vi "Video read with led for drums.vi"() -> ()   [LabVIEW 2009]
uses:
  <vilib>/vision/Image Controls.llb/IMAQ Image.ctl
  <vilib>/Instr/_visa.llb/VISA Configure Serial Port (Instr).vi
  <vilib>/Analysis/3filter.llb/Filter Passband Type.ctl
  <vilib>/Analysis/3filter.llb/Butterworth Filter (DBL).vi
  <vilib>/vision/NI_Vision_Development_Module.lvlib
  <vilib>/Analysis/NI_AALBase.lvlib
panel:
  in  "Mask":T1 {"Contours"."Type" items=["No Selection", "Point", "Line", "Rectangle", "Oval", "Polygon", "Freehand Region", "Annulus", "Unused2", "Unused3", "Broken Line", "Freehand Line", "Rotated Rectangle"]}
  out "Image 2":T2(plugin-control)
  out "Red Line":T1={"Global Rectangle"=[300, 297, 320, 380], "Contours"=[{"ID"=enum."External", "Type"=2, "Coordinates"=[300, 379, 319, 297]}]} {"Contours"."Type" items=["No Selection", "Point", "Line", "Rectangle", "Oval", "Polygon", "Freehand Region", "Annulus", "Unused2", "Unused3", "Broken Line", "Freehand Line", "Rotated Rectangle"]}
  in  "Red Line":T1={"Global Rectangle"=[300, 297, 320, 380], "Contours"=[{"ID"=enum."External", "Type"=2, "Coordinates"=[300, 379, 319, 297]}]} {"Contours"."Type" items=["No Selection", "Point", "Line", "Rectangle", "Oval", "Polygon", "Freehand Region", "Annulus", "Unused2", "Unused3", "Broken Line", "Freehand Line", "Rotated Rectangle"]}
  out "Waveform Red":dbl[](graph)
  out "LED Red":bool
  in  "sampling 4":dbl=1.0 format="%0.2f"
  in  "high 4":dbl=60.0 format="%0.2f"
  in  "low  4":dbl=0.12500000000000006 format="%0.4f"
  out "Green Line":T1={"Global Rectangle"=[406, 309, 423, 383], "Contours"=[{"ID"=enum."External", "Type"=2, "Coordinates"=[422, 382, 406, 309]}]} {"Contours"."Type" items=["No Selection", "Point", "Line", "Rectangle", "Oval", "Polygon", "Freehand Region", "Annulus", "Unused2", "Unused3", "Broken Line", "Freehand Line", "Rotated Rectangle"]}
  in  "Blue Line":T1={"Global Rectangle"=[374, 278, 383, 377], "Contours"=[{"ID"=enum."External", "Type"=2, "Coordinates"=[382, 376, 374, 278]}]} {"Contours"."Type" items=["No Selection", "Point", "Line", "Rectangle", "Oval", "Polygon", "Freehand Region", "Annulus", "Unused2", "Unused3", "Broken Line", "Freehand Line", "Rotated Rectangle"]}
  in  "Green Line":T1={"Global Rectangle"=[406, 309, 423, 383], "Contours"=[{"ID"=enum."External", "Type"=2, "Coordinates"=[422, 382, 406, 309]}]} {"Contours"."Type" items=["No Selection", "Point", "Line", "Rectangle", "Oval", "Polygon", "Freehand Region", "Annulus", "Unused2", "Unused3", "Broken Line", "Freehand Line", "Rotated Rectangle"]}
  in  "low  3":dbl=0.12500000000000006 format="%0.4f"
  out "Waveform Green":dbl[](graph)
  out "LED Green":bool
  in  "sampling 3":dbl=1.0 format="%0.2f"
  in  "high 3":dbl=60.0 format="%0.2f"
  in  "Yellow Line":T1={"Global Rectangle"=[342, 292, 349, 377], "Contours"=[{"ID"=enum."External", "Type"=2, "Coordinates"=[342, 376, 348, 292]}]} {"Contours"."Type" items=["No Selection", "Point", "Line", "Rectangle", "Oval", "Polygon", "Freehand Region", "Annulus", "Unused2", "Unused3", "Broken Line", "Freehand Line", "Rotated Rectangle"]}
  out "Blue Line":T1={"Global Rectangle"=[168, 264, 180, 378], "Contours"=[{"ID"=enum."External", "Type"=2, "Coordinates"=[168, 377, 179, 264]}]} {"Contours"."Type" items=["No Selection", "Point", "Line", "Rectangle", "Oval", "Polygon", "Freehand Region", "Annulus", "Unused2", "Unused3", "Broken Line", "Freehand Line", "Rotated Rectangle"]}
  out "cluster":T3
  in  "baud rate (9600)":u32=9600
  in  "VISA resource name":refnum<visa-resource-name>
  out "number":u32
  out "decimal integer string":string
  out "Image Dst Out":T2
  out "Yellow Line":T1={"Global Rectangle"=[243, 262, 261, 384], "Contours"=[{"ID"=enum."External", "Type"=2, "Coordinates"=[260, 383, 243, 262]}]} {"Contours"."Type" items=["No Selection", "Point", "Line", "Rectangle", "Oval", "Polygon", "Freehand Region", "Annulus", "Unused2", "Unused3", "Broken Line", "Freehand Line", "Rotated Rectangle"]}
  in  "low  2":dbl=0.12500000000000006 format="%0.4f"
  in  "high 2":dbl=60.0 format="%0.2f"
  in  "sampling 2":dbl=1.0 format="%0.2f"
  out "LED Yellow":bool
  out "Waveform Yellow":dbl[](graph)
  in  "playtime":dbl=30.0
  out "Frame Number":i32
  in  "Frame Start":i32=2400
  out "LED BLUE":bool
  in  "low":dbl=0.12500000000000006 format="%0.4f"
  out "Waveform Blue":dbl[](graph)
  in  "high":dbl=60.0 format="%0.2f"
  in  "sampling":dbl=1.0 format="%0.2f"
  in  "stop":bool
  in  "AVI Path":path
  # "BLUE"
  # "YELLOW"
  # "GREEN"
  # "RED"
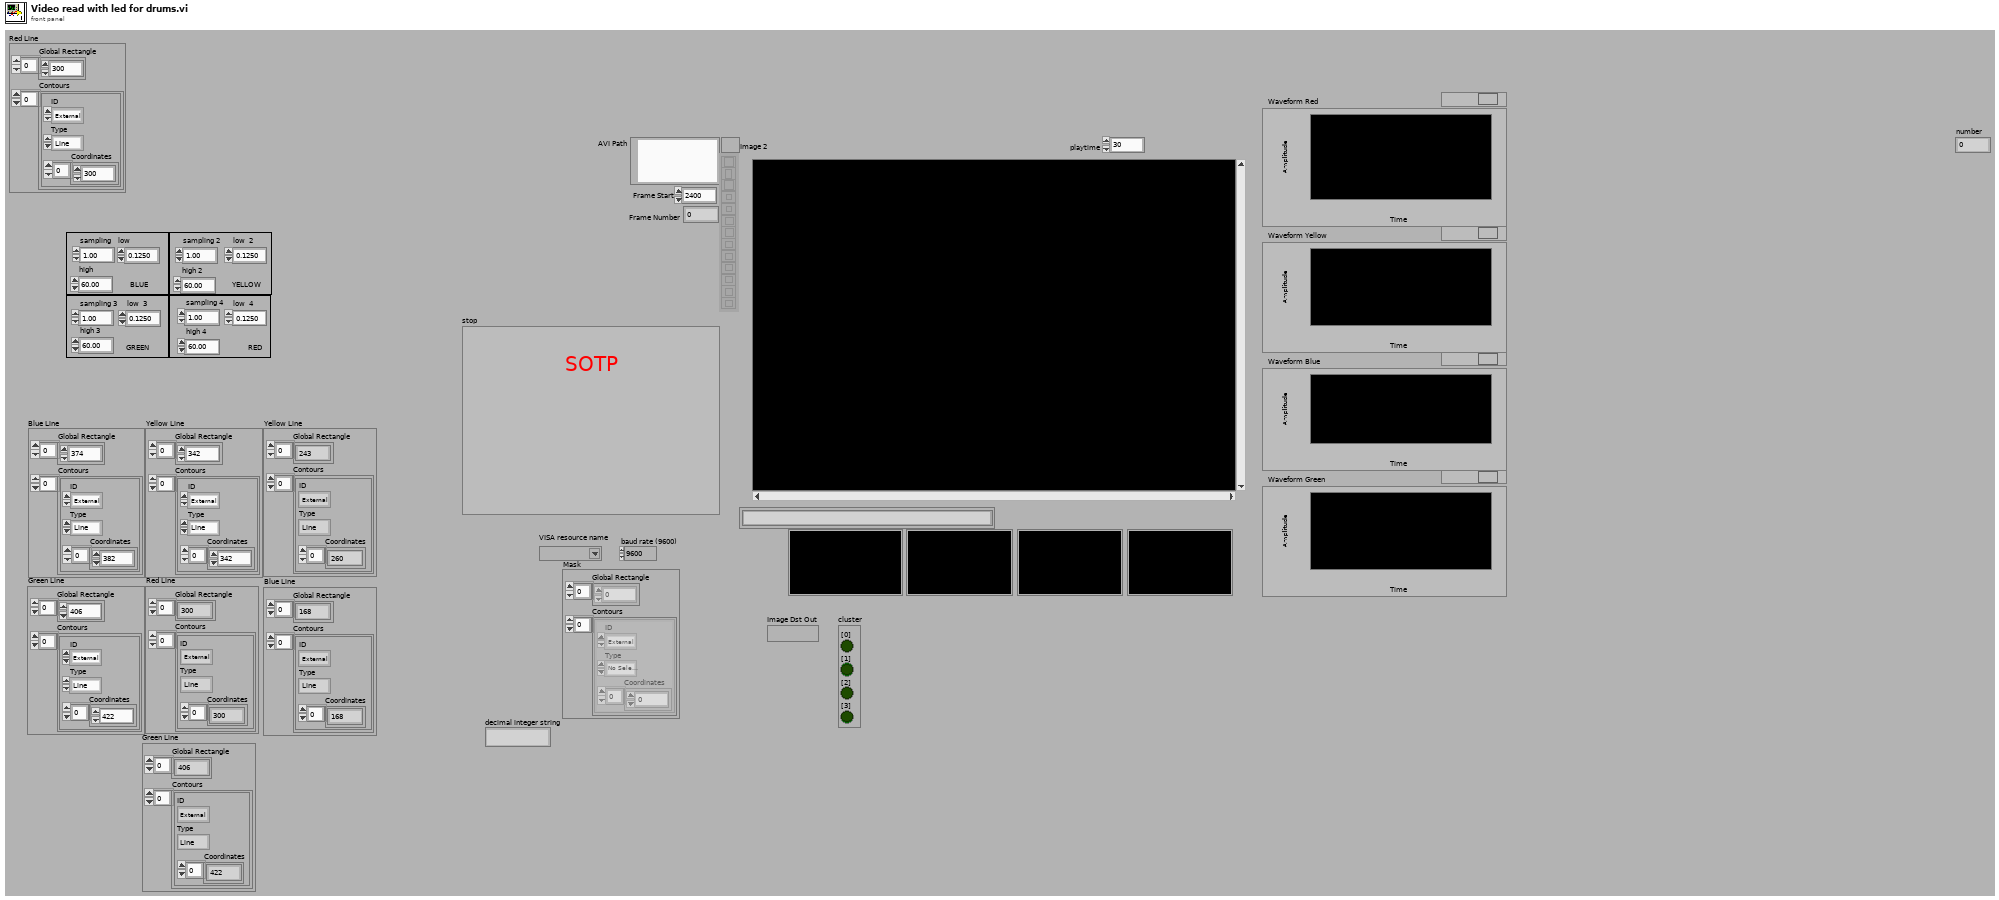
[diagram p1: front panel]
types:
  T1 = cluster{"Global Rectangle":i32[], "Contours":cluster{"ID":enum32{"External", "Internal"}, "Type":u32, "Coordinates":i32[]}[]}
  T2 = typedef "IMAQ Image.ctl" = refnum<image>
  T3 = cluster{"[0]":bool, "[1]":bool, "[2]":bool, "[3]":bool, "[4]":bool, "[5]":bool, "[6]":bool, "[7]":bool, "[8]":bool}
  T4 = typedef "NI_AALBase.lvlib/Filter Passband Type.ctl" = enum32{"Lowpass", "Highpass", "Bandpass", "Bandstop"}
  T5 = cluster{"Left":i32, "Top":i32, "Right":i32, "Bottom":i32}
  T6 = typedef "Image Type" = u32
  T7 = typedef "AviRefnum.ctl" = refnum<k1>
  T8 = cluster{"ID":enum32{"External", "Internal"}, "Type":u32, "Coordinates":i32[]}[]
  T9 = cluster{"ID":enum32{"External", "Internal"}, "Type":u32, "Coordinates":i32[]}
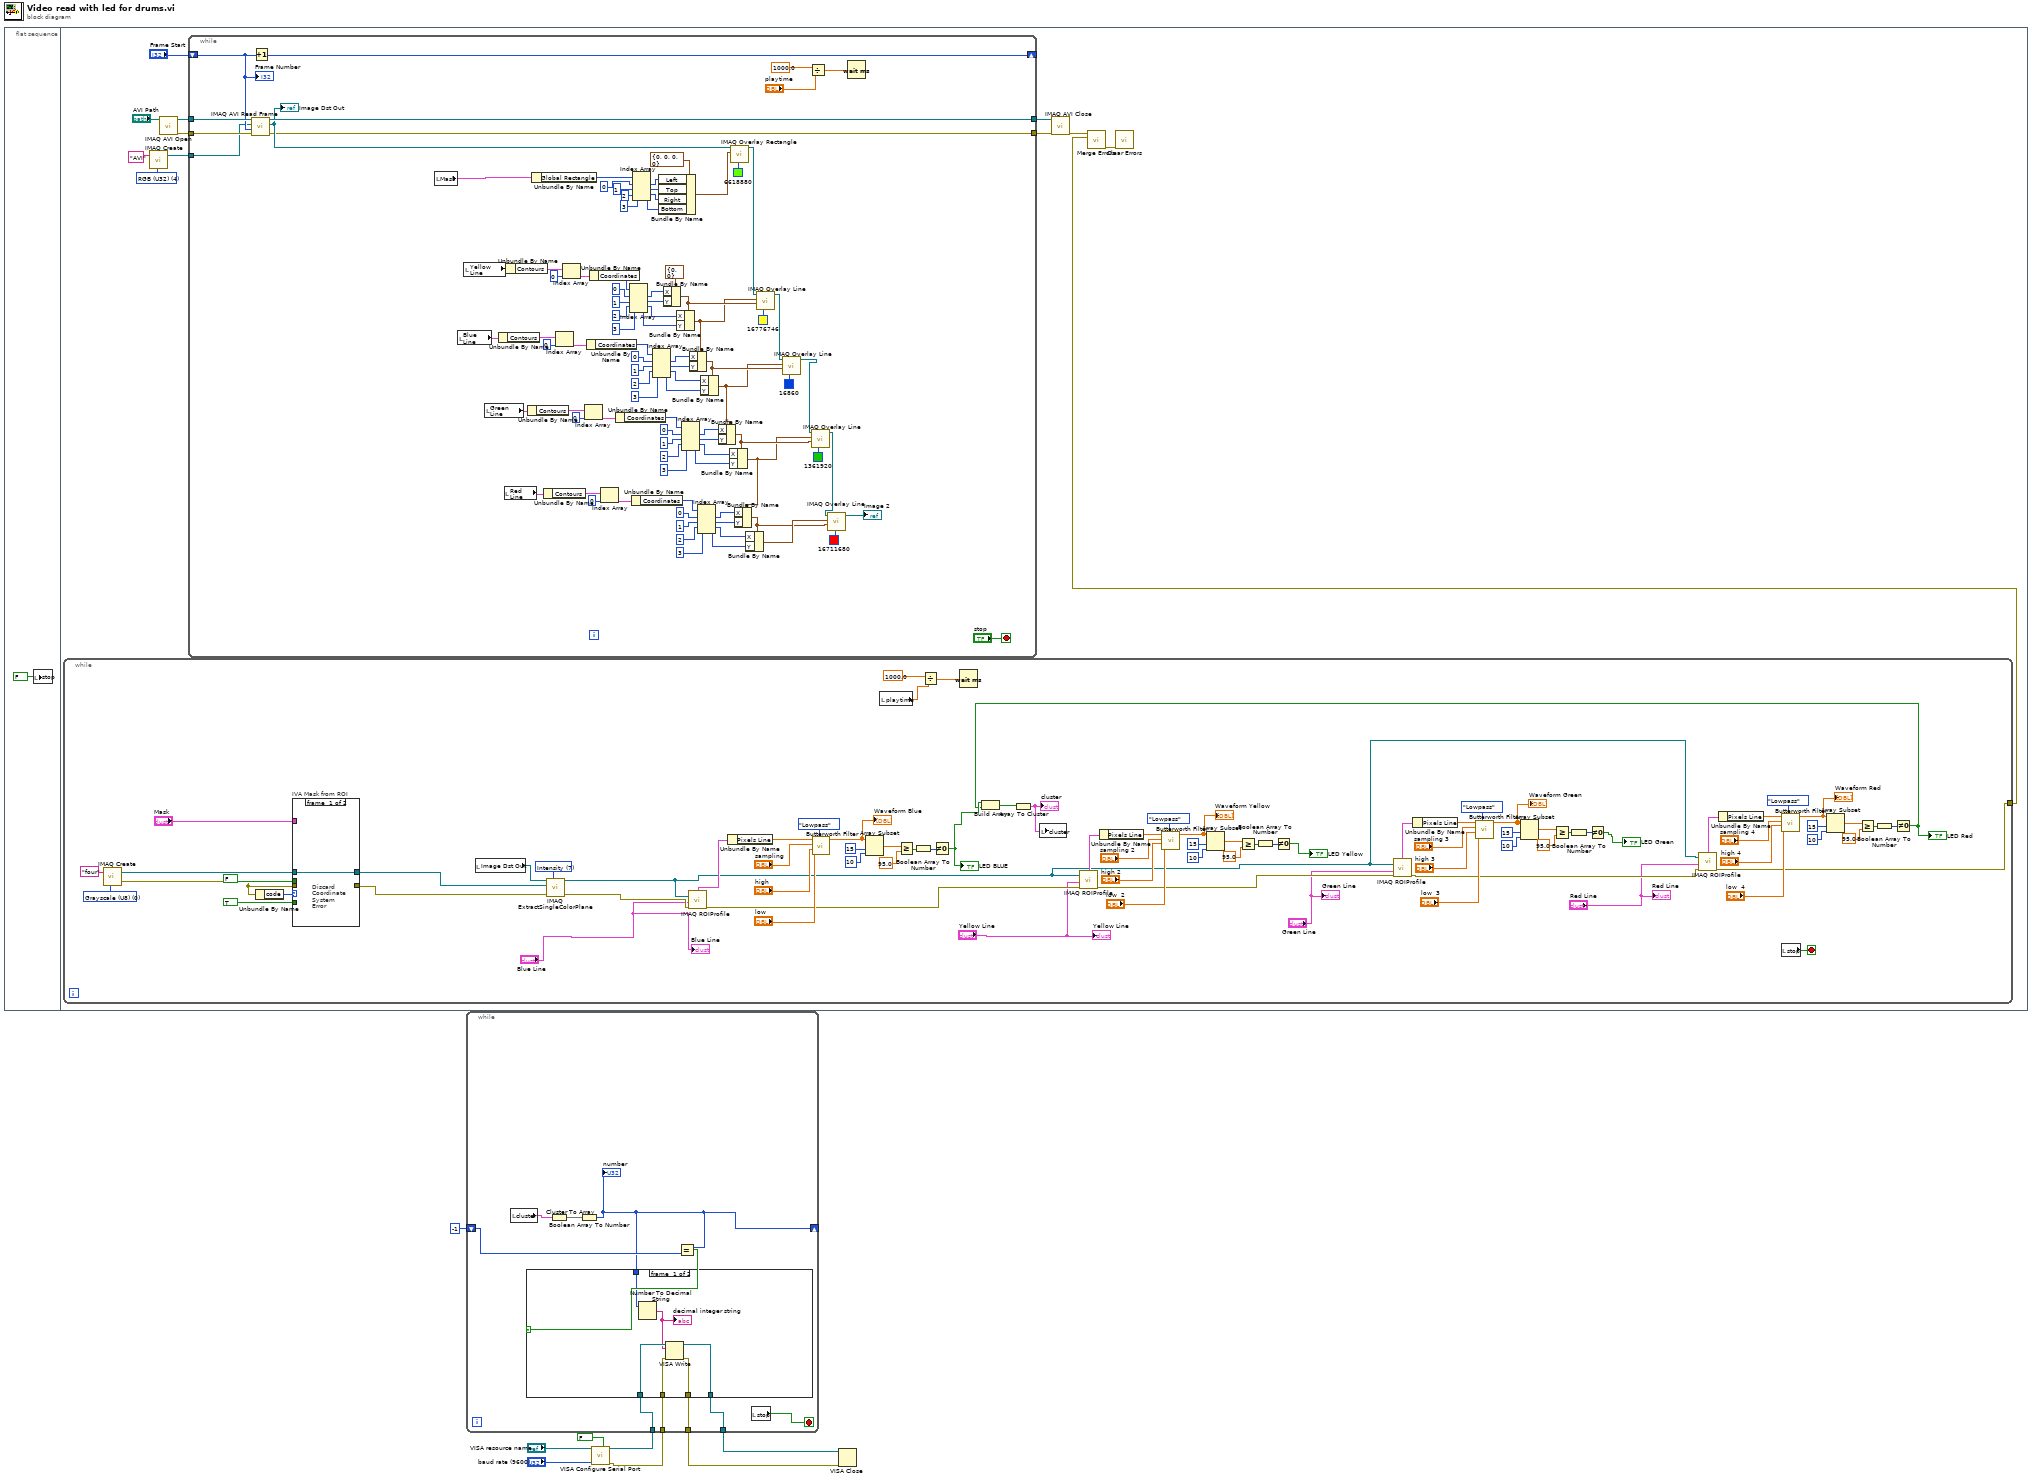
[diagram p0: block diagram]
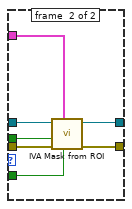
[diagram p3: hidden frame]
diagram:
  n1 = flat-sequence {
    frame #0 {
      n2 = local write "stop"(FALSE ("stop")) -> ()
    }
    frame #1 {
      w13 = T6 4 items=["Grayscale (U8)", "Grayscale (I16)", "Grayscale (SGL)", "Complex (CSG)", "RGB (U32)", "HSL (U32)", "RGB (U64)", "Grayscale (U16)"] ("Image Type")
      n3 = while {
        tunnel: [w34] -> w10
        stop <- w104 stop-if-true
        w75 = T6 0 items=["Grayscale (U8)", "Grayscale (I16)", "Grayscale (SGL)", "Complex (CSG)", "RGB (U32)", "HSL (U32)", "RGB (U64)", "Grayscale (U16)"] ("Image Type")
        w105 = 7 items=["Red", "Green", "Blue", "Hue", "Saturation", "Luminance", "Value", "Intensity"] ("Color Plane")
        n4 = call "IMAQ Create"("Image Name"="four", "Image Type"=w75) -> ("New Image"=w26:T2, "error out"=w27:errorcluster)  [unwired: 3 in]
        n5 = Unbundle By Name(w27) -> ("code"=w31:i32)
        n6 = case "IVA Mask from ROI" shown="Default" w31 {
          tunnel: "Mask" -> [_ w113]
          tunnel: TRUE ("Shrink") -> [_ w112]
          tunnel: w26 -> [w106 w111]
          tunnel: w27 -> [_ w110]
          tunnel: [_ w109] -> w28
          tunnel: [w106 w108] -> w24
          tunnel: FALSE ("Out / In") -> [_ w107]
          frame #0 {
            # "Discard\nCoordinate\nSystem\nError"
          }
          frame #1 {
            n7 = call <vilib>:"IVA Mask from ROI.vi"("Shrink"=w112, "ROI Descriptor"=w113, "error in (no error)"=w110, "Out / In"=w107, "Image Src"=w111) -> ("error out"=w109:errorcluster, "Image Out"=w108:T2)  [unwired: 5 out]
          }
        }
        n8 = local read "Image Dst Out"() -> (w76:T2)
        n9 = call "IMAQ ExtractSingleColorPlane"("Color Plane"=w105, "error in (no error)"=w28, "Image Dst"=w24, "Image Src"=w76) -> ("error out"=w68:errorcluster, "Image Dst Out"=w32:T2)  [unwired: 6 out]
        n10 = call "IMAQ ROIProfile"("error in (no error)"=w68, "ROI Descriptor"="Blue Line", "Image"=w32) -> ("error out"=w69:errorcluster, "ROI Graph"=w67:cluster{"x0":sgl, "dx":sgl, "Pixels Line":sgl[]})  [unwired: 4 out]
        n11 = Unbundle By Name(w67) -> ("Pixels Line"=w102:sgl[])
        n12 = call-poly <vilib>:"Butterworth Filter.vi"("filter type"=Filter_Passband_Type."Lowpass", "low cutoff freq: fl"="low", "high cutoff freq: fh"="high", "sampling freq: fs"="sampling", "X"=w102) -> ("Filtered X"=w50:dbl[])  [unwired: 3 in, 1 out]
        "Waveform Blue" <- w50
        n13 = Array Subset(array=w50, index=15, length=10) -> (w96:dbl[])
        n14 = local read "playtime"() -> (w90:dbl)
        n15 = Greater Or Equal?(x=w96, y=95.0) -> (x >= y?=w94:bool[])
        n16 = Boolean Array To Number(Boolean array=w94) -> (number=w91:u32)
        n17 = Divide(x=1000.0, y=w90) -> (x/y=w93:dbl)
        n18 = Not Equal To 0?(x=w91) -> (x != 0?=w70:bool)
        "LED BLUE" <- w70
        n19 = Wait (ms)(milliseconds to wait=w93) -> ()  [unwired: 1 out]
        n20 = call "IMAQ ROIProfile"("error in (no error)"=w69, "ROI Descriptor"="Yellow Line", "Image"=w32) -> ("error out"=w53:errorcluster, "ROI Graph"=w79:cluster{"x0":sgl, "dx":sgl, "Pixels Line":sgl[]})  [unwired: 4 out]
        n21 = Unbundle By Name(w79) -> ("Pixels Line"=w82:sgl[])
        n22 = call-poly <vilib>:"Butterworth Filter.vi"("filter type"=Filter_Passband_Type."Lowpass", "low cutoff freq: fl"="low  2", "high cutoff freq: fh"="high 2", "sampling freq: fs"="sampling 2", "X"=w82) -> ("Filtered X"=w78:dbl[])  [unwired: 3 in, 1 out]
        "Waveform Yellow" <- w78
        n23 = Array Subset(array=w78, index=15, length=10) -> (w87:dbl[])
        n24 = Greater Or Equal?(x=w87, y=95.0) -> (x >= y?=w85:bool[])
        n25 = Boolean Array To Number(Boolean array=w85) -> (number=w84:u32)
        n26 = Not Equal To 0?(x=w84) -> (x != 0?=→"LED Yellow":bool)
        n27 = call "IMAQ ROIProfile"("error in (no error)"=w53, "ROI Descriptor"="Green Line", "Image"=w32) -> ("error out"=w35:errorcluster, "ROI Graph"=w64:cluster{"x0":sgl, "dx":sgl, "Pixels Line":sgl[]})  [unwired: 4 out]
        n28 = Unbundle By Name(w64) -> ("Pixels Line"=w61:sgl[])
        n29 = call-poly <vilib>:"Butterworth Filter.vi"("filter type"=Filter_Passband_Type."Lowpass", "low cutoff freq: fl"="low  3", "high cutoff freq: fh"="high 3", "sampling freq: fs"="sampling 3", "X"=w61) -> ("Filtered X"=w65:dbl[])  [unwired: 3 in, 1 out]
        "Waveform Green" <- w65
        n30 = Array Subset(array=w65, index=15, length=10) -> (w56:dbl[])
        n31 = Greater Or Equal?(x=w56, y=95.0) -> (x >= y?=w58:bool[])
        n32 = Boolean Array To Number(Boolean array=w58) -> (number=w59:u32)
        n33 = Not Equal To 0?(x=w59) -> (x != 0?=→"LED Green":bool)
        n34 = call "IMAQ ROIProfile"("error in (no error)"=w35, "ROI Descriptor"="Red Line", "Image"=w32) -> ("error out"=w34:errorcluster, "ROI Graph"=w37:cluster{"x0":sgl, "dx":sgl, "Pixels Line":sgl[]})  [unwired: 4 out]
        n35 = Unbundle By Name(w37) -> ("Pixels Line"=w40:sgl[])
        n36 = call-poly <vilib>:"Butterworth Filter.vi"("filter type"=Filter_Passband_Type."Lowpass", "low cutoff freq: fl"="low  4", "high cutoff freq: fh"="high 4", "sampling freq: fs"="sampling 4", "X"=w40) -> ("Filtered X"=w36:dbl[])  [unwired: 3 in, 1 out]
        "Waveform Red" <- w36
        n37 = local read "stop"() -> (w104:bool)
        n38 = Array Subset(array=w36, index=15, length=10) -> (w45:dbl[])
        n39 = Greater Or Equal?(x=w45, y=95.0) -> (x >= y?=w43:bool[])
        n40 = Boolean Array To Number(Boolean array=w43) -> (number=w42:u32)
        n41 = Not Equal To 0?(x=w42) -> (x != 0?=w22:bool)
        "LED Red" <- w22
        n42 = Build Array(w70, w22) -> (w73:bool[])
        n43 = Array To Cluster(array=w73) -> (cluster=w72:T3)
        "cluster" <- w72
        n44 = local write "cluster"(w72) -> ()
        "Yellow Line" <- "Yellow Line"
        "Blue Line" <- "Blue Line"
        "Green Line" <- "Green Line"
        "Red Line" <- "Red Line"
      }
      n45 = call "IMAQ Create"("Image Name"="AVI", "Image Type"=w13) -> ("New Image"=w11:T2)  [unwired: 3 in, 1 out]
      n46 = call "IMAQ AVI Open"("AVI Path"="AVI Path") -> ("error out"=w18:errorcluster, "Avi Refnum"=w19:T7)  [unwired: 9 in]
      n47 = while {
        tunnel: w19 -> [w208]
        tunnel: w18 -> [w156]
        tunnel: [w207] -> w20
        shift-right: [w202] -> _
        shift-left: "Frame Start" -> [w201]
        tunnel: [w152] -> w14
        tunnel: w11 -> [w151]
        stop <- "stop" stop-if-true
        n48 = call "IMAQ AVI Read Frame"("error in (no error)"=w156, "Frame Number"=w201, "Image"=w151, "Avi Refnum"=w208) -> ("error out"=w152:errorcluster, "Image Out"=w153:T2, "Avi Refnum (duplicate)"=w207:T7)  [unwired: 4 in, 1 out]
        "Image Dst Out" <- w153
        n49 = Increment(x=w201) -> (x+1=w202:i32)
        n50 = local read "Mask"() -> (w114:T1)
        n51 = local read "Blue Line"() -> (w155:T1)
        n52 = local read "Yellow Line"() -> (w154:T1)
        n53 = local read "Green Line"() -> (w150:T1)
        n54 = Unbundle By Name(w155) -> ("Contours"=w168:T8)
        n55 = local read "Red Line"() -> (w117:T1)
        n56 = Unbundle By Name(w154) -> ("Contours"=w183:T8)
        n57 = Unbundle By Name(w150) -> ("Contours"=w140:T8)
        n58 = Unbundle By Name(w114) -> ("Global Rectangle"=w197:i32[])
        n59 = Unbundle By Name(w117) -> ("Contours"=w127:T8)
        n60 = Index Array(array=w168, index=0) -> (element=w167:T9)
        n61 = Index Array(array=w183, index=0) -> (element=w185:T9)
        n62 = Index Array(array=w140, index=0) -> (element=w141:T9)
        n63 = Unbundle By Name(w167) -> ("Coordinates"=w166:i32[])
        n64 = Unbundle By Name(w185) -> ("Coordinates"=w186:i32[])
        n65 = Index Array(array=w127, index=0) -> (element=w126:T9)
        n66 = Unbundle By Name(w141) -> ("Coordinates"=w142:i32[])
        n67 = Index Array(array=w186, index #1=0 ("index"), index #2=1 ("index"), index #3=2 ("index"), index #4=3 ("index")) -> (element #1=w178:i32, element #2=w179:i32, element #3=w180:i32, element #4=w181:i32)
        n68 = Unbundle By Name(w126) -> ("Coordinates"=w125:i32[])
        n69 = Index Array(array=w197, index #1=0 ("index"), index #2=1 ("index"), index #3=2 ("index"), index #4=3 ("index")) -> (element #1=w196:i32, element #2=w195:i32, element #3=w194:i32, element #4=w193:i32)
        n70 = Index Array(array=w166, index #1=0 ("index"), index #2=1 ("index"), index #3=2 ("index"), index #4=3 ("index")) -> (element #1=w165:i32, element #2=w171:i32, element #3=w170:i32, element #4=w169:i32)
        n71 = Bundle By Name(cluster=T5 {"Left"=0, "Top"=0, "Right"=0, "Bottom"=0} ("Rectangle"), "Left"=w196, "Top"=w195, "Right"=w194, "Bottom"=w193) -> (w199:T5)
        n72 = Bundle By Name(cluster=cluster{"X":i32, "Y":i32} {"X"=0, "Y"=0} ("End Point"), "X"=w178, "Y"=w179) -> (w187:cluster{"X":i32, "Y":i32})
        n73 = Bundle By Name(cluster=w187, "X"=w180, "Y"=w181) -> (w158:cluster{"X":i32, "Y":i32})
        n74 = Index Array(array=w142, index #1=0 ("index"), index #2=1 ("index"), index #3=2 ("index"), index #4=3 ("index")) -> (element #1=w143:i32, element #2=w137:i32, element #3=w138:i32, element #4=w139:i32)
        n75 = Bundle By Name(cluster=w158, "X"=w165, "Y"=w171) -> (w172:cluster{"X":i32, "Y":i32})
        n76 = Index Array(array=w125, index #1=0 ("index"), index #2=1 ("index"), index #3=2 ("index"), index #4=3 ("index")) -> (element #1=w124:i32, element #2=w130:i32, element #3=w129:i32, element #4=w128:i32)
        n77 = Bundle By Name(cluster=w172, "X"=w170, "Y"=w169) -> (w135:cluster{"X":i32, "Y":i32})
        n78 = Bundle By Name(cluster=w135, "X"=w143, "Y"=w137) -> (w134:cluster{"X":i32, "Y":i32})
        n79 = Bundle By Name(cluster=w134, "X"=w138, "Y"=w139) -> (w116:cluster{"X":i32, "Y":i32})
        n80 = call "IMAQ Overlay Rectangle"("Color"=u32 6618880, "Rectangle"=w199, "Image"=w153) -> ("Image Out"=w173:T2)  [unwired: 7 in, 1 out]
        n81 = Bundle By Name(cluster=w116, "X"=w124, "Y"=w130) -> (w132:cluster{"X":i32, "Y":i32})
        n82 = Bundle By Name(cluster=w132, "X"=w129, "Y"=w128) -> (w133:cluster{"X":i32, "Y":i32})
        n83 = call "IMAQ Overlay Line"("Color"=u32 16776746, "End Point"=w187, "Start Point"=w158, "Image"=w173) -> ("Image Out"=w163:T2)  [unwired: 6 in, 1 out]
        n84 = call "IMAQ Overlay Line"("Color"=u32 16860, "End Point"=w172, "Start Point"=w135, "Image"=w163) -> ("Image Out"=w136:T2)  [unwired: 6 in, 1 out]
        n85 = Divide(x=1000.0, y="playtime") -> (x/y=w205:dbl)
        n86 = call "IMAQ Overlay Line"("Color"=u32 1361920, "End Point"=w134, "Start Point"=w116, "Image"=w136) -> ("Image Out"=w115:T2)  [unwired: 6 in, 1 out]
        n87 = call "IMAQ Overlay Line"("Color"=u32 16711680, "End Point"=w132, "Start Point"=w133, "Image"=w115) -> ("Image Out"=→"Image 2":T2)  [unwired: 6 in, 1 out]
        n88 = Wait (ms)(milliseconds to wait=w205) -> ()  [unwired: 1 out]
        "Frame Number" <- w201
      }
      n89 = call "IMAQ AVI Close"("error in (no error)"=w14, "Avi Refnum"=w20) -> ("error out"=w16:errorcluster)  [unwired: 9 in]
      n90 = call <vilib>:"Merge Errors.vi"("error in 2 (no error)"=w10, "error in 1 (no error)"=w16) -> ("error out"=w15:errorcluster)  [unwired: 5 in]
      n91 = call <vilib>:"Clear Errors.vi"("error in (no error)"=w15) -> ()  [unwired: 6 in, 1 out]
    }
  }
  n92 = call-poly "VISA Configure Serial Port"("VISA resource name"="VISA resource name", "Enable Termination\nChar (T)"=FALSE ("Enable Termination\nChar (T)"), "baud rate (9600)"="baud rate (9600)") -> ("VISA resource name out"=w7:refnum<visa-resource-name>, "error out"=w2:errorcluster)  [unwired: 11 in]
  n93 = while {
    shift-right: [w212] -> _
    shift-left: -1 -> [w218]
    tunnel: w7 -> [w216]
    tunnel: [w215] -> w6
    tunnel: w2 -> [w214]
    tunnel: [w213] -> w1
    stop <- w209 stop-if-true
    n94 = local read "cluster"() -> (w210:T3)
    n95 = Cluster To Array(cluster=w210) -> (array=w211:bool[])
    n96 = Boolean Array To Number(Boolean array=w211) -> (number=w212:u32)
    "number" <- w212
    n97 = Equal?(x=w212, y=w218) -> (x = y?=w217:bool)
    n98 = case shown="False" w217 {
      tunnel: w216 -> [w224 w226]
      tunnel: [w223 w226] -> w215
      tunnel: w212 -> [w221 _]
      tunnel: w214 -> [w220 w225]
      tunnel: [w219 w225] -> w213
      frame #0 {
        n99 = Number To Decimal String(number=w221) -> (decimal integer string=w222:string)  [unwired: 1 in]
        "decimal integer string" <- w222
        n100 = VISA Write(VISA resource name=w224, write buffer=w222, error in (no error)=w220) -> (VISA resource name out=w223:refnum<visa-resource-name>, error out=w219:errorcluster)  [unwired: 1 out]
      }
      frame #1 {
      }
    }
    n101 = local read "stop"() -> (w209:bool)
  }
  n102 = VISA Close(VISA resource name=w6, error in (no error)=w1) -> ()  [unwired: 1 out]
